vi "Analyze Debug Event.vi"(8 "error in (no error)":errorcluster, 10 "Debug Data.lvclass":refnum<class "Debug Data.lvclass">, 11 "Debug State Analyzer In":refnum<class "Debug State Analyzer.lvclass">) -> (0 "error out":errorcluster, 3 "Debug State Analyzer Out":refnum<class "Debug State Analyzer.lvclass">)   [LabVIEW 2020, in "Debug State Analyzer.lvclass"]
uses:
  Debug State Analyzer.lvclass
  Debug Data/Debug Data.lvclass
  Debug Data/Debug Data.lvclass/Debug Data.ctl
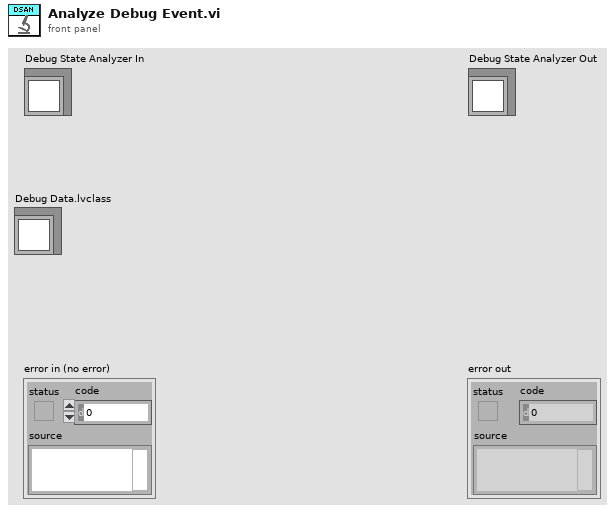
[diagram p1: front panel]
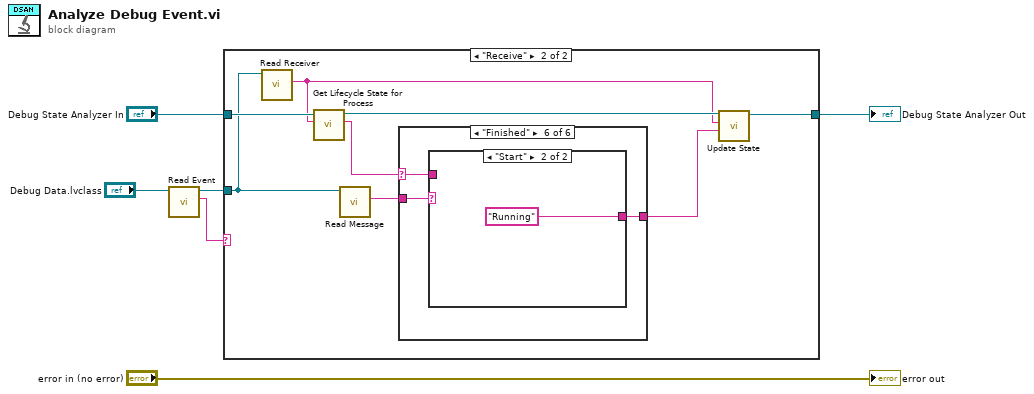
[diagram p0: block diagram]
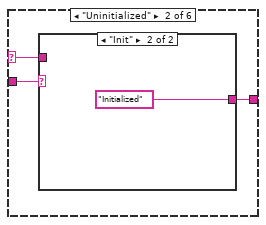
[diagram p4: hidden frame]
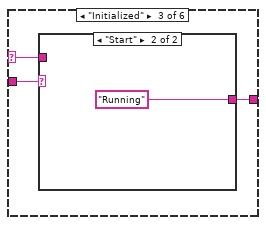
[diagram p6: hidden frame]
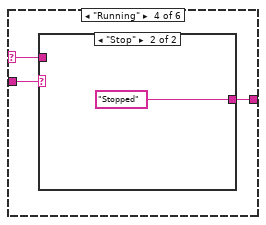
[diagram p8: hidden frame]
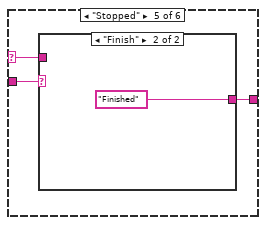
[diagram p10: hidden frame]
diagram:
  n1 = call "Read Event.vi"("Debug Data in"="Debug Data.lvclass") -> ("Event"=w4:string, "Debug Data out"=w3:refnum<class "Debug Data.lvclass">)  [unwired: 9 in]
  n2 = case shown="\"Receive\"" w4 {
    tunnel: w3 -> [_ w13]
    tunnel: "Debug State Analyzer In" -> [w7 w15]
    tunnel: [w7 w10] -> w1
    frame Default {
    }
    frame "Receive" {
      n3 = call "Read Receiver.vi"("Debug Data In"=w13) -> ("Receiver"=w9:string)  [unwired: 9 in, 1 out]
      n4 = call "Get Lifecycle State for Process.vi"("Process"=w9, "Debug State Analyzer In"=w15) -> ("Lifecycle State"=w14:string, "Debug State Analyzer Out"=w11:refnum<class "Debug State Analyzer.lvclass">)  [unwired: 8 in]
      n5 = call "Read Message.vi"("Debug Data in"=w13) -> ("Message"=w12:string)  [unwired: 8 in, 2 out]
      n6 = case shown="\"Finished\"" w14 {
        selector: w14 -> [w16 w17 w22 w27 w32 w37]
        tunnel: w12 -> [_ w19 w24 w29 w34 w39]
        tunnel: [w16 w18 w23 w28 w33 w38] -> w8
        frame Default {
        }
        frame "Uninitialized" {
          n7 = case shown="\"Init\"" w19 {
            tunnel: [w20 "Initialized"] -> w18
            tunnel: w17 -> [w20 _]
            frame Default {
            }
            frame "Init" {
            }
          }
        }
        frame "Initialized" {
          n8 = case shown="\"Start\"" w24 {
            tunnel: [w25 "Running"] -> w23
            tunnel: w22 -> [w25 _]
            frame Default {
            }
            frame "Start" {
            }
          }
        }
        frame "Running" {
          n9 = case shown="\"Stop\"" w29 {
            tunnel: [w30 "Stopped"] -> w28
            tunnel: w27 -> [w30 _]
            frame Default {
            }
            frame "Stop" {
            }
          }
        }
        frame "Stopped" {
          n10 = case shown="\"Finish\"" w34 {
            tunnel: [w35 "Finished"] -> w33
            tunnel: w32 -> [w35 _]
            frame Default {
            }
            frame "Finish" {
            }
          }
        }
        frame "Finished" {
          n11 = case shown="\"Start\"" w39 {
            tunnel: [w40 "Running"] -> w38
            tunnel: w37 -> [w40 _]
            frame Default {
            }
            frame "Start" {
            }
          }
        }
      }
      n12 = call "Update State.vi"("New State"=w8, "Process"=w9, "Debug State Analyzer In"=w11) -> ("Debug State Analyzer Out"=w10:refnum<class "Debug State Analyzer.lvclass">)  [unwired: 8 in]
    }
  }
  "Debug State Analyzer Out" <- w1
  "error out" <- "error in (no error)"
